vi "remove.vi"(8 "error in (no error)":errorcluster, 10 "Composite Employee.lvclass":refnum<class "Composite Employee.lvclass">, 11 "Composite Employee in":refnum<class "Composite Employee.lvclass">) -> (0 "error out":errorcluster, 3 "Composite Employee out":refnum<class "Composite Employee.lvclass">)   [LabVIEW 2016, in "Composite Employee.lvclass"]
uses:
  Composite Employee.lvclass
  C:/Users/Felipe/Desktop/LabVIEW OOP Design Patters Folder/LabVIEW OOP Design Patters Folder/Composite Pattern/Employee Class/Employee.lvclass
  Composite Employee.lvclass/Composite Employee.ctl
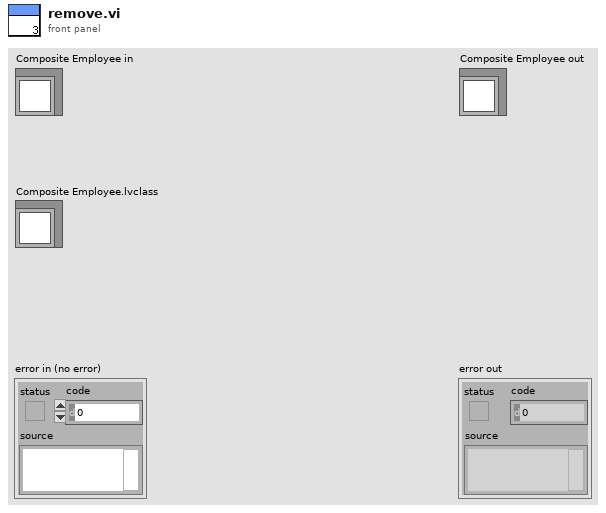
[diagram p1: front panel]
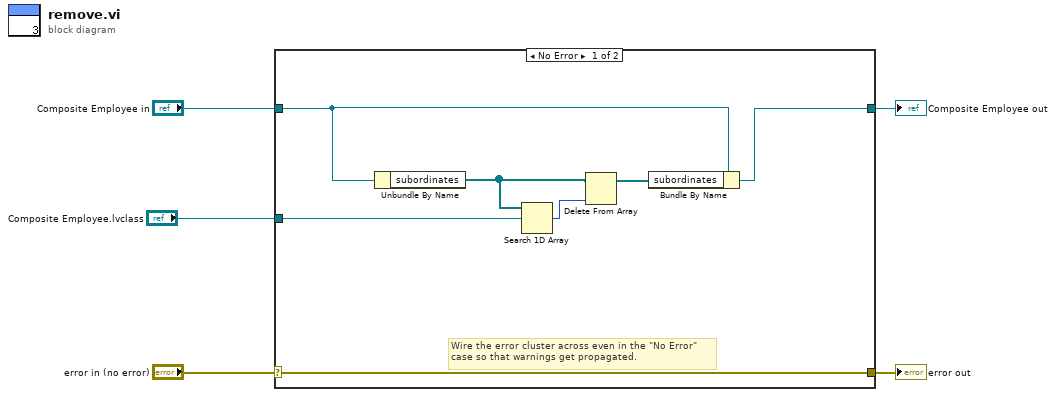
[diagram p0: block diagram]
diagram:
  n1 = case shown="No Error" "error in (no error)" {
    selector: "error in (no error)" -> [w12 w14]
    tunnel: [w12 w14] -> w4
    tunnel: [w10 w13] -> w2
    tunnel: "Composite Employee in" -> [w11 w13]
    tunnel: "Composite Employee.lvclass" -> [w9 _]
    frame No Error {
      # "Wire the error cluster across even in the \"No Error\"\ncase so that warnings get propagated."
      n2 = Unbundle By Name(w11) -> ("subordinates"=w6:refnum<class "Employee.lvclass">[])
      n3 = Search 1D Array(1D array=w6, element=w9) -> (index of element=w8:i32)  [unwired: 1 in]
      n4 = Delete From Array(array=w6, index=w8) -> (array with subset deleted=w7:refnum<class "Employee.lvclass">[])  [unwired: 1 in, 1 out]
      n5 = Bundle By Name(cluster=w11, "subordinates"=w7) -> (w10:refnum<class "Composite Employee.lvclass">)
    }
    frame Error {
    }
  }
  "error out" <- w4
  "Composite Employee out" <- w2
